vi "imageQ_create_return_queue.vi"(1 "Queue Name":string="ImageQCameraImages") -> (0 "queue out":refnum<queue>)   [LabVIEW 2015]
uses:
  <vilib>/vision/Image Controls.llb/IMAQ Image.ctl
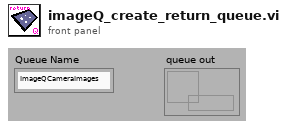
[diagram p1: front panel]
types:
  T1 = typedef "IMAQ Image.ctl" = refnum<image>
  T2 = cluster{"Camera Image":T1, "ROI":u64[], "Timestamp/us":u64}
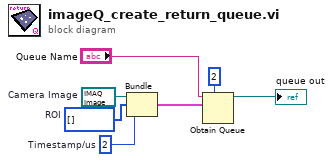
[diagram p0: block diagram]
diagram:
  w5 = u64 2  # Timestamp/us
  w4 = u64[] []  # ROI
  w3 = T1 refnum  # Camera Image
  n1 = Bundle("Camera Image"=w3, "ROI"=w4, "Timestamp/us"=w5) -> (w6:T2)  [unwired: 1 in]
  n2 = Obtain Queue(max queue size (-1, unlimited)=2, name (unnamed)="Queue Name", element data type=w6) -> (queue out=→"queue out":refnum<queue>)  [unwired: 2 in, 2 out]
